vi "CommandToScript.vi"(8 "error in (no error)":errorcluster, 9 "Feedrate In":dbl, 10 "Position In":dbl, 11 "Command In":string="IDLE") -> (0 "error out":errorcluster, 3 "AeroBasic Template Out":string)   [LabVIEW 2013, in "Aerotech_Soloist.lvclass"]
uses:
  Aerotech_Soloist.lvclass
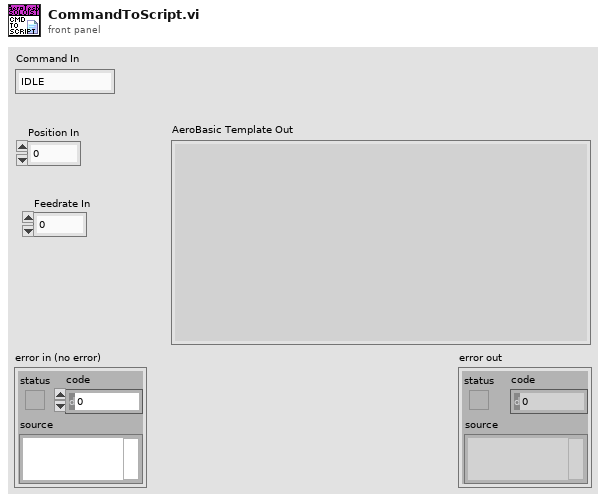
[diagram p1: front panel]
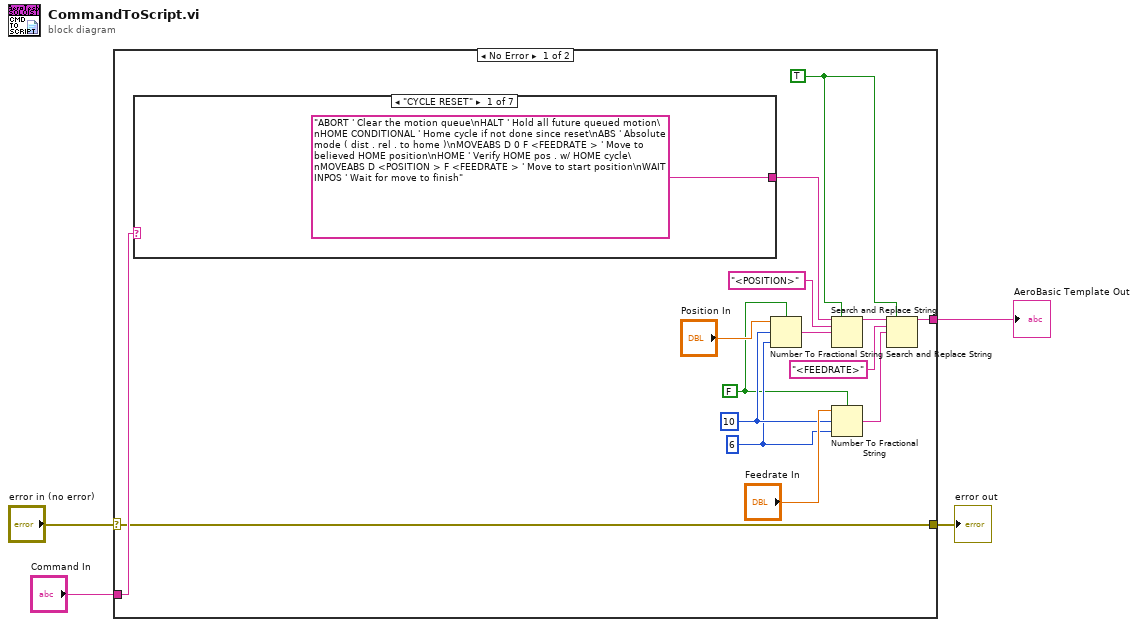
[diagram p0: block diagram]
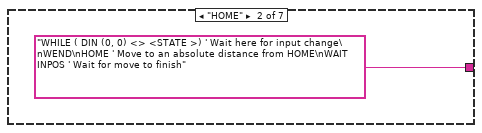
[diagram p2: hidden frame]
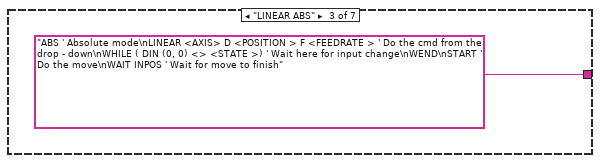
[diagram p3: hidden frame]
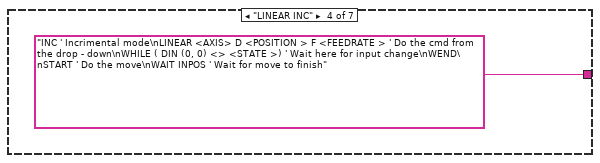
[diagram p4: hidden frame]
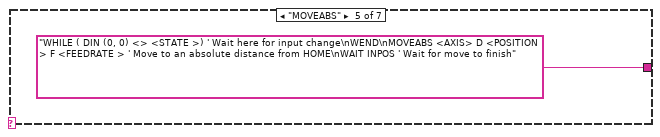
[diagram p5: hidden frame]
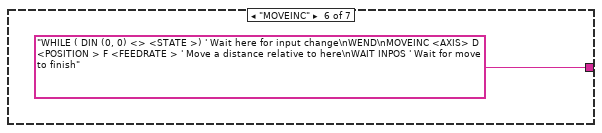
[diagram p6: hidden frame]
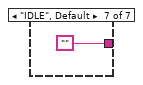
[diagram p7: hidden frame]
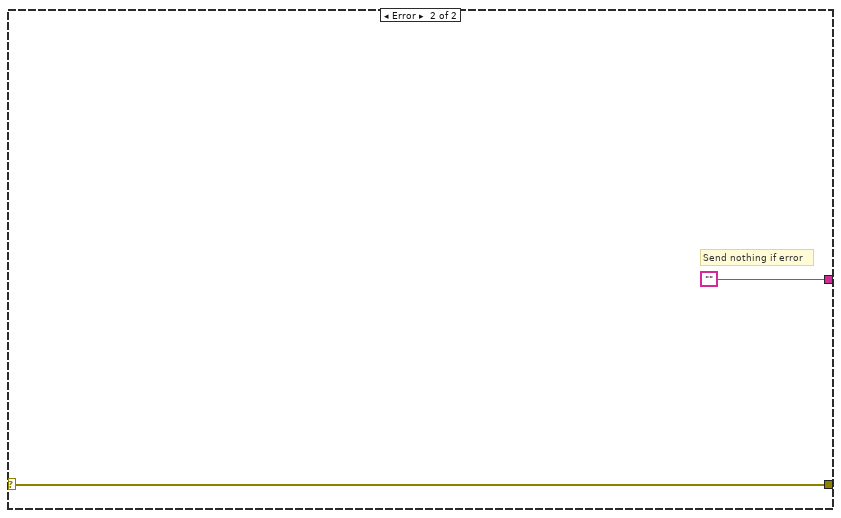
[diagram p8: hidden frame]
diagram:
  n1 = case shown="No Error" "error in (no error)" {
    selector: "error in (no error)" -> [w7 w28]
    tunnel: [w7 w28] -> w3
    tunnel: [w6 ""] -> w2
    tunnel: "Command In" -> [w19 _]
    frame No Error {
      w9 = FALSE ("use system decimal point (T)")
      w14 = TRUE ("replace all? (F)")
      w10 = i16 6 ("precision (6)")
      w11 = i16 10 ("width (-)")
      n2 = case shown="\"CYCLE RESET\"" w19 {
        tunnel: ["ABORT ' Clear the motion queue\nHALT ' Hold all future queued motion\nHOME CONDITIONAL ' Home cycle if not done since reset\nABS ' Absolute mode ( dist . rel . to home )\nMOVEABS D 0 F <FEEDRATE > ' Move to believed HOME position\nHOME ' Verify HOME pos . w/ HOME cycle\nMOVEABS D <POSITION > F <FEEDRATE > ' Move to start position\nWAIT INPOS ' Wait for move to finish" "WHILE ( DIN (0, 0) <> <STATE >) ' Wait here for input change\nWEND\nHOME ' Move to an absolute distance from HOME\nWAIT INPOS ' Wait for move to finish" "ABS ' Absolute mode\nLINEAR <AXIS> D <POSITION > F <FEEDRATE > ' Do the cmd from the drop - down\nWHILE ( DIN (0, 0) <> <STATE >) ' Wait here for input change\nWEND\nSTART ' Do the move\nWAIT INPOS ' Wait for move to finish" "INC ' Incrimental mode\nLINEAR <AXIS> D <POSITION > F <FEEDRATE > ' Do the cmd from the drop - down\nWHILE ( DIN (0, 0) <> <STATE >) ' Wait here for input change\nWEND\nSTART ' Do the move\nWAIT INPOS ' Wait for move to finish" "WHILE ( DIN (0, 0) <> <STATE >) ' Wait here for input change\nWEND\nMOVEABS <AXIS> D <POSITION > F <FEEDRATE > ' Move to an absolute distance from HOME\nWAIT INPOS ' Wait for move to finish" "WHILE ( DIN (0, 0) <> <STATE >) ' Wait here for input change\nWEND\nMOVEINC <AXIS> D <POSITION > F <FEEDRATE > ' Move a distance relative to here\nWAIT INPOS ' Wait for move to finish" ""] -> w15
        frame "CYCLE RESET" {
        }
        frame "HOME" {
        }
        frame "LINEAR ABS" {
        }
        frame "LINEAR INC" {
        }
        frame "MOVEABS" {
        }
        frame "MOVEINC" {
        }
        frame "IDLE", Default {
        }
      }
      n3 = Number To Fractional String(use system decimal point (T)=w9, number="Position In", width (-)=w11, precision (6)=w10) -> (F-format string=w17:string)
      n4 = Search and Replace String(replace all?=w14, input string=w15, search string="<POSITION>", replace string=w17) -> (result string=w5:string)  [unwired: 4 in, 3 out]
      n5 = Number To Fractional String(use system decimal point (T)=w9, number="Feedrate In", width (-)=w11, precision (6)=w10) -> (F-format string=w8:string)
      n6 = Search and Replace String(replace all?=w14, input string=w5, search string="<FEEDRATE>", replace string=w8) -> (result string=w6:string)  [unwired: 4 in, 3 out]
    }
    frame Error {
      # "Send nothing if error"
    }
  }
  "error out" <- w3
  "AeroBasic Template Out" <- w2
